vi "csv_control_00.vi"() -> ()   [LabVIEW 2024]
panel:
  in  "Test_Value":dbl
  in  "Test_ID":string
  in  "SN":string
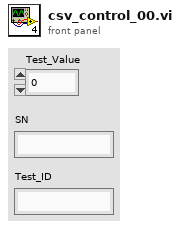
[diagram p1: front panel]
types:
  T1 = enum16{"open", "replace", "create", "open or create", "replace or create", "replace or create with confirmation"}
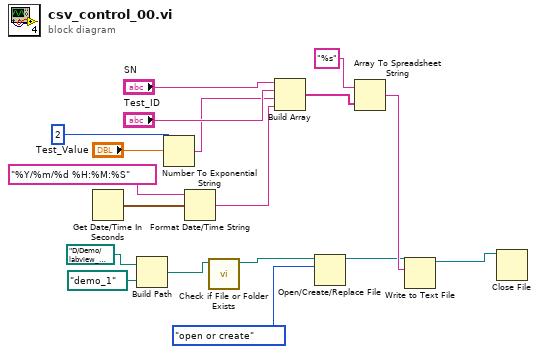
[diagram p0: block diagram]
diagram:
  n1 = Get Date/Time In Seconds() -> (seconds since 1Jan1904=w12:timestamp)
  n2 = Build Path(base path=path "D:/Demo/labview_demo/data&docu" ("基路径"), name or relative path=path "demo_1" ("名称或相对路径")) -> (appended path=w18:path)
  n3 = Number To Exponential String(number="Test_Value", precision (6)=i16 2 ("精度(6)")) -> (E-format string=w13:string)  [unwired: 2 in]
  n4 = Format Date/Time String(time format string (%c)="%Y/%m/%d %H:%M:%S" ("时间格式字符串(%c)"), seconds (now)=w12) -> (date/time string=w10:string)  [unwired: 1 in]
  n5 = call <vilib>:"Check if File or Folder Exists.vi"("path"=w18) -> ("dup path"=w17:path)  [unwired: 8 in, 2 out]
  n6 = Build Array("SN", "Test_ID", w13, w10) -> (w9:string[])
  n7 = Open/Create/Replace File(file path (use dialog)=w17, operation (0:open)=T1."open or create" ("操作(0:open)")) -> (refnum out=w6:refnum<file>)  [unwired: 4 in, 2 out]
  n8 = Array To Spreadsheet String(array=w9, 3:"%s" ("格式字符串")) -> (spreadsheet string=w8:string)  [unwired: 1 in]
  n9 = Write to Text File(file (use dialog)=w6, text=w8) -> (refnum out=w5:refnum<file>)  [unwired: 2 in, 2 out]
  n10 = Close File(refnum=w5) -> ()  [unwired: 1 in, 2 out]
